vi "Find All Paths.vi"(7 "path":i32[](array[numeric]), 8 "error in (no error)":errorcluster, 9 "End Vertex":i32, 10 "Start Vertex":i32, 11 "Graph In":refnum<class "Graph.lvclass">) -> (0 "error out":errorcluster, 2 "paths":i32[][](array[numeric]), 3 "Graph out":refnum<class "Graph.lvclass">)   [LabVIEW 2013, in "Graph.lvclass"]
uses:
  Graph.lvclass
  Graph.lvclass/Graph.ctl
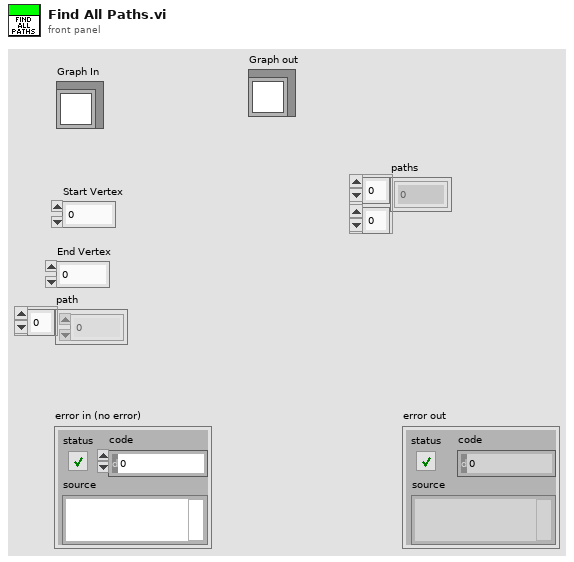
[diagram p1: front panel]
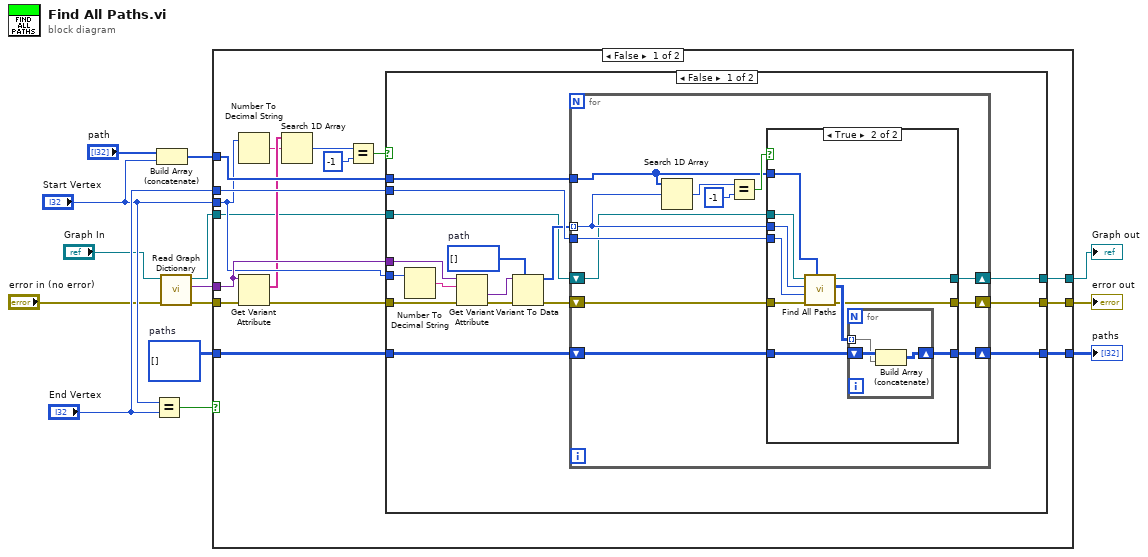
[diagram p0: block diagram]
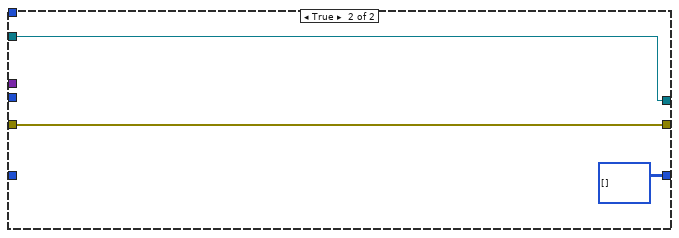
[diagram p3: hidden frame]
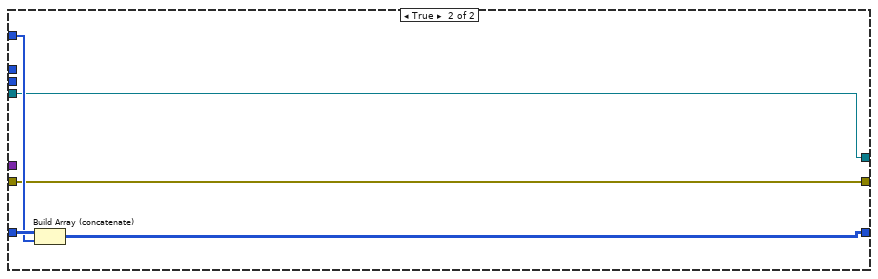
[diagram p4: hidden frame]
diagram:
  w10 = i32[][] []  # paths
  n1 = Equal?(x="Start Vertex", y="End Vertex") -> (x = y?=w11:bool)
  n2 = Build Array (concatenate)("path", "Start Vertex") -> (w7:i32[])
  n3 = call "Read Graph Dictionary.vi"("error in (no error)"="error in (no error)", "Graph in"="Graph In") -> ("error out"=w3:errorcluster, "Graph Dictionary"=w6:variant, "Graph out"=w2:refnum<class "Graph.lvclass">)  [unwired: 7 in]
  n4 = case shown="False" w11 {
    tunnel: w7 -> [w30 w81]
    tunnel: [w29 w79] -> w14
    tunnel: "Start Vertex" -> [w23 _]
    tunnel: "End Vertex" -> [w28 _]
    tunnel: [w27 w80] -> w13
    tunnel: w10 -> [w26 w82]
    tunnel: w6 -> [w24 _]
    tunnel: w3 -> [w17 w79]
    tunnel: w2 -> [w16 w78]
    tunnel: [w15 w78] -> w1
    frame False {
      n5 = Number To Decimal String(number=w23) -> (decimal integer string=w21:string)  [unwired: 1 in]
      n6 = Get Variant Attribute(Variant=w24, error in=w17) -> (names=w22:string[], error out=w25:errorcluster)  [unwired: 2 in, 2 out]
      n7 = Search 1D Array(1D array=w22, element=w21) -> (index of element=w20:i32)  [unwired: 1 in]
      n8 = Equal?(x=w20, y=-1) -> (x = y?=w18:bool)
      n9 = case shown="False" w18 {
        tunnel: w30 -> [w33 _]
        tunnel: [w46 w77] -> w29
        tunnel: w23 -> [w45 _]
        tunnel: w28 -> [w44 _]
        tunnel: w25 -> [w37 w77]
        tunnel: [w36 i32[][] [] ("paths")] -> w27
        tunnel: w26 -> [w35 _]
        tunnel: w24 -> [w34 _]
        tunnel: w16 -> [w32 w75]
        tunnel: [w31 w75] -> w15
        frame False {
          w40 = i32[] []  # path
          n10 = Number To Decimal String(number=w45) -> (decimal integer string=w43:string)  [unwired: 1 in]
          n11 = Get Variant Attribute(Variant=w34, name=w43, error in=w37) -> (value=w42:variant, error out=w41:errorcluster)  [unwired: 1 in, 2 out]
          n12 = Variant To Data(error in=w41, type=w40, Variant=w42) -> (data=w39:i32[], error out=w38:errorcluster)
          n13 = for {
            tunnel: w39 -> [w53] mode=indexing
            tunnel: w33 -> [w49]
            shift-right: [w54] -> w46
            shift-left: w38 -> [w55]
            tunnel: w44 -> [w52]
            shift-right: [w50] -> w36
            shift-left: w35 -> [w51]
            shift-right: [w47] -> w31
            shift-left: w32 -> [w48]
            n14 = Search 1D Array(1D array=w49, element=w53) -> (index of element=w57:i32)  [unwired: 1 in]
            n15 = Equal?(x=w57, y=-1) -> (x = y?=w56:bool)
            n16 = case shown="True" w56 {
              tunnel: w55 -> [w61 w68]
              tunnel: [w61 w67] -> w54
              tunnel: w53 -> [_ w66]
              tunnel: w52 -> [_ w65]
              tunnel: w51 -> [w60 w71]
              tunnel: [w60 w69] -> w50
              tunnel: w49 -> [_ w64]
              tunnel: w48 -> [w59 w63]
              tunnel: [w59 w62] -> w47
              frame False {
              }
              frame True {
                n17 = call "Find All Paths.vi"("path"=w64, "error in (no error)"=w68, "End Vertex"=w65, "Start Vertex"=w66, "Graph In"=w63) -> ("error out"=w67:errorcluster, "paths"=w70:i32[][], "Graph out"=w62:refnum<class "Graph.lvclass">)  [unwired: 4 in]
                n18 = for {
                  shift-right: [w74] -> w69
                  shift-left: w71 -> [w73]
                  tunnel: w70 -> [w72] mode=indexing
                  n19 = Build Array (concatenate)(w73, w72) -> (w74:i32[][])
                }
              }
            }
          }
        }
        frame True {
        }
      }
    }
    frame True {
      n20 = Build Array (concatenate)(w82, w81) -> (w80:i32[][])
    }
  }
  "error out" <- w14
  "paths" <- w13
  "Graph out" <- w1
